vi "Get Node by NodePath(No Traverse).vi"(8 "error in (no error)":errorcluster caption="错误输入（无错误）", 10 "NodePath":string, 11 "PanelLinkNode 输入":refnum<class "PanelLinkNode.lvclass"> caption="DNL_LabVIEW Object in") -> (0 "error out":errorcluster caption="错误输出", 2 "Node*":refnum<data-value>, 3 "PanelLinkNode 输出":refnum<class "PanelLinkNode.lvclass"> caption="DNL_LabVIEW Object out")   [LabVIEW 2013, in "PanelLinkNode.lvclass"]
uses:
  PanelLinkNode.lvclass
  PanelObject/PanelObject.lvclass
  PanelLinkNode.lvclass/PanelLinkNode.ctl
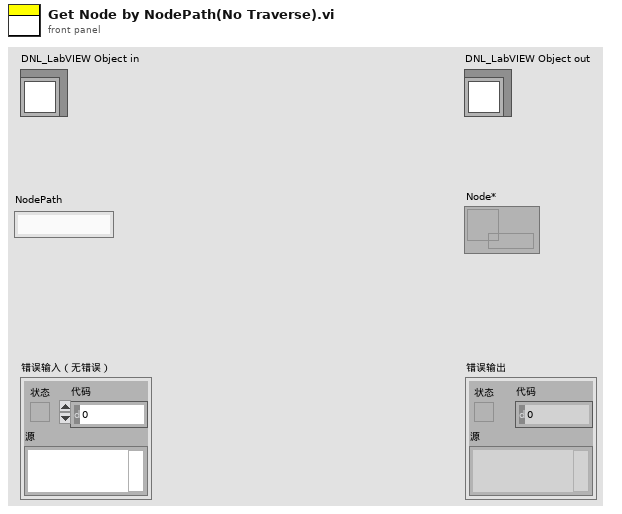
[diagram p1: front panel]
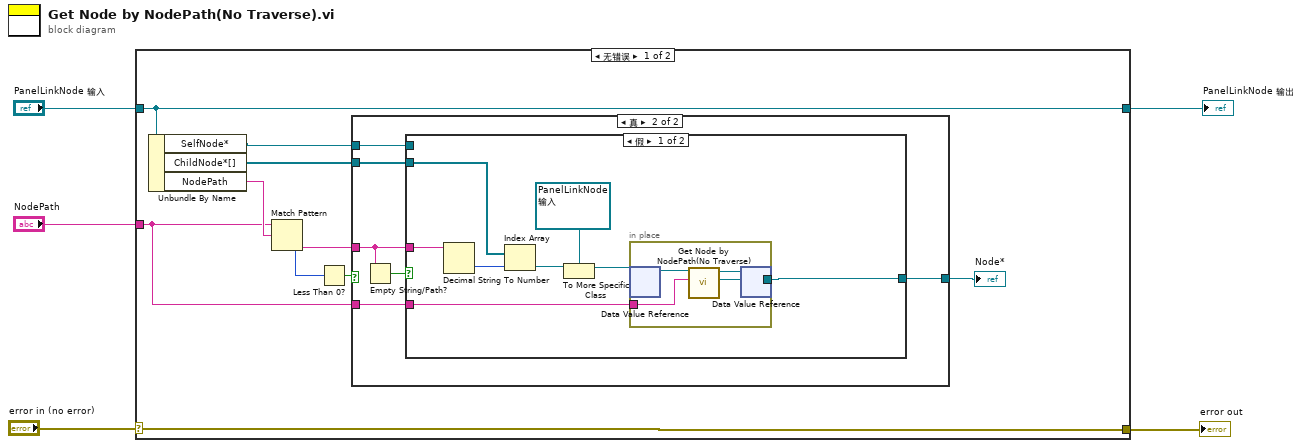
[diagram p0: block diagram]
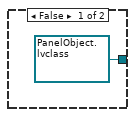
[diagram p2: hidden frame]
diagram:
  n1 = case shown="无错误" "error in (no error)" {
    selector: "error in (no error)" -> [w15 w37]
    tunnel: [w15 w37] -> w4
    tunnel: [w9 w36] -> w2
    tunnel: "PanelLinkNode 输入" -> [w9 w36]
    tunnel: "NodePath" -> [w8 _]
    frame No Error {
      n2 = Unbundle By Name(w9) -> ("SelfNode*"=w7:refnum<data-value>, "ChildNode*[]"=w10:refnum<data-value>[], "NodePath"=w14:string)
      n3 = Match Pattern(string=w8, regular expression=w14) -> (after substring=w11:string, offset past match=w13:i32)  [unwired: 1 in, 2 out]
      n4 = Less Than 0?(x=w13) -> (x < 0?=w12:bool)
      n5 = case shown="真" w12 {
        tunnel: w11 -> [_ w20]
        tunnel: w10 -> [_ w21]
        tunnel: w8 -> [_ w19]
        tunnel: w7 -> [_ w18]
        tunnel: [refnum<data-value> refnum ("SelfNode*") w17] -> w6
        frame False {
        }
        frame True {
          n6 = Empty String/Path?(string/path=w20) -> (empty?=w22:bool)
          n7 = case shown="假" w22 {
            tunnel: w21 -> [w29 _]
            tunnel: w20 -> [w30 _]
            tunnel: w19 -> [w24 _]
            tunnel: w18 -> [_ w35]
            tunnel: [w23 w35] -> w17
            frame False {
              n8 = Decimal String To Number(string=w30) -> (number=w28:i32)  [unwired: 2 in, 1 out]
              n9 = Index Array(array=w29, index=w28) -> (element=w27:refnum<data-value>)
              n10 = To More Specific Class(target class=refnum<data-value> refnum ("数据值引用"), reference=w27) -> (specific class reference=w25:refnum<data-value>)  [unwired: 1 in, 1 out]
              n11 = in-place {
                in-place-border: w24 -> [w32]
                in-place-border: [w31] -> w23
                n12 = in-place-dvr #1(w25) -> (w34:refnum<class "PanelLinkNode.lvclass">)  [unwired: 1 out]
                n13 = call-dynamic "Get Node by NodePath(No Traverse).vi"("NodePath"=w32, "PanelLinkNode 输入"=w34) -> ("Node*"=w31:refnum<data-value>, "PanelLinkNode 输出"=w33:refnum<class "PanelLinkNode.lvclass">)  [unwired: 7 in, 1 out]
                n14 = in-place-dvr #1(w33) -> ()  [unwired: 2 out]
              }
            }
            frame True {
            }
          }
        }
      }
      "Node*" <- w6
    }
    frame Error {
    }
  }
  "error out" <- w4
  "PanelLinkNode 输出" <- w2
